vi "pulse_train.vi"() -> ()   [LabVIEW 2018]
panel:
  out "Array":bool[](array[boolean])
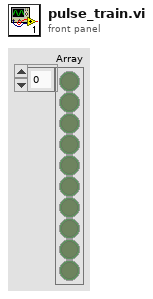
[diagram p1: front panel]
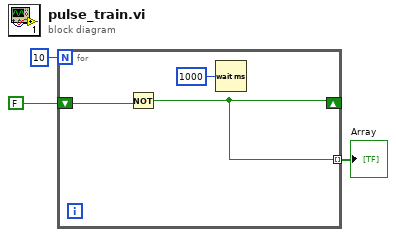
[diagram p0: block diagram]
diagram:
  n1 = for {
    N: 10 -> [_]
    shift-right: [w4] -> _
    shift-left: FALSE -> [w6]
    tunnel: [w4] -> w1 mode=indexing
    n2 = Not(x=w6) -> (.not. x?=w4:bool)
    n3 = Wait (ms)(milliseconds to wait=u32 1000) -> ()  [unwired: 1 out]
  }
  "Array" <- w1
